vi "WriteOVASprdshtFile.vi"(0 "Source Matrix":u8(ring) items=["A", "B", "C"], 1 "Graph Data to Output":bool[](array[boolean]), 2 "Filter?":bool=TRUE, 3 "Resolution BW (GHz)":dbl=5.0 format="%.2f", 4 "RBW Units for Output":u8(ring) items=["pm", "GHz"], 5 "error in (no error)":errorcluster, 6 "Output Spreadsheet File Path":path=path "C:/ss.txt", 7 "Cursor Indices":u32[](array[numeric])=[0, 0], 8 "Device Descriptor":string, 9 "chanwidthstr":string) -> (19 "error out":errorcluster)   [LabVIEW 2024]
uses:
  OVA32.dll
panel:
  # "Used for LPD & QPD"
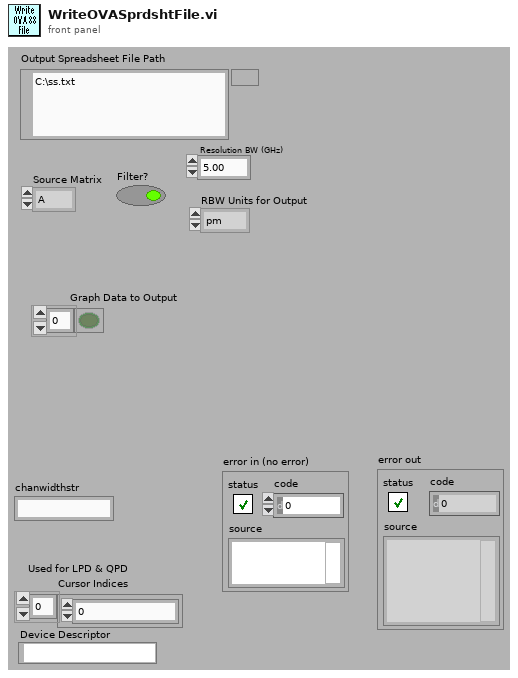
[diagram p1: front panel]
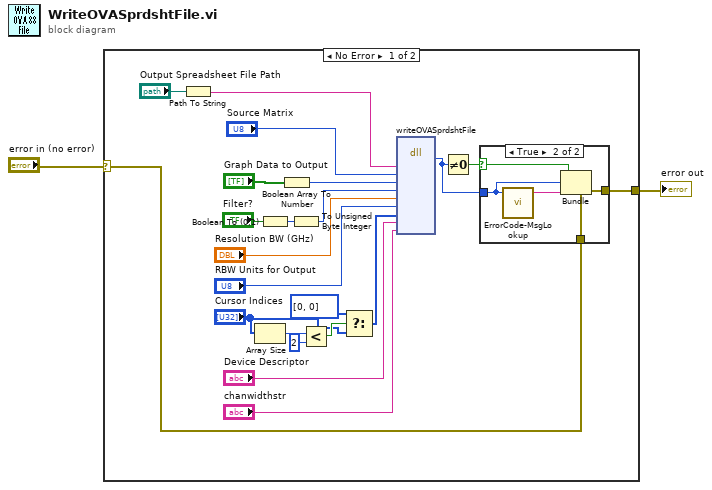
[diagram p0: block diagram]
diagram:
  n1 = case shown="No Error" "error in (no error)" {
    selector: "error in (no error)" -> [w13 w31]
    tunnel: [w12 w31] -> w1
    frame No Error {
      n2 = Path To String(path="Output Spreadsheet File Path") -> (string=w23:string)
      n3 = Array Size(array="Cursor Indices") -> (size(s)=w11:i32)
      n4 = Boolean To (0,1)(Boolean="Filter?") -> (0, 1=w19:i16)
      n5 = Boolean Array To Number(Boolean array="Graph Data to Output") -> (number=w21:u32)
      n6 = To Unsigned Byte Integer(number=w19) -> (unsigned 8bit integer=w18:u8)
      n7 = Less?(x=w11, y=2) -> (x < y?=w8:bool)
      n8 = Select(t=u32[] [0, 0] ("Cursor Indices"), s=w8, f="Cursor Indices") -> (s? t:f=w6:u32[])
      n9 = dll-call lib="OVA32.dll" fn="writeOVASprdshtFile" label="writeOVASprdshtFile()"("SSFileName"=w23, "measMatrix"="Source Matrix", "graphsFlag"=w21, "filter"=w18, "filterRBW"="Resolution BW (GHz)", "outRBWunits"="RBW Units for Output", "indices"=w6, "descriptor"="Device Descriptor", "chanwidthstr"="chanwidthstr") -> (w14:i32)  [unwired: 12 in, 2 out]
      n10 = Not Equal To 0?(x=w14) -> (x != 0?=w15:bool)
      n11 = case shown="True" w15 {
        selector: w15 -> [_ w27]
        tunnel: w14 -> [_ w28]
        tunnel: w13 -> [w25 w30]
        tunnel: [w25 w26] -> w12
        frame False {
        }
        frame True {
          n12 = call "ErrorCode-MsgLookup.vi"("DLL Return Code"=w28) -> ("Error String"=w29:string)  [unwired: 2 in, 2 out]
          n13 = Bundle(cluster=w30, "status"=w27, "code"=w28, "source"=w29) -> (w26:errorcluster)
        }
      }
    }
    frame Error {
    }
  }
  "error out" <- w1
